vi "DecodifyFrequency.vi"   [LabVIEW 2017, in "AODControl.lvlib"]
uses:
  AODControl.lvlib
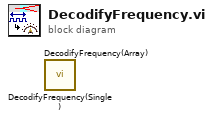
[diagram p0: block diagram]
diagram:
  n1 = call "DecodifyFrequency(Single).vi"() -> ()  [unwired: 1 in, 1 out]
  n2 = call "DecodifyFrequency(Array).vi"() -> ()  [unwired: 1 in, 1 out]
